vi "SiggenSetFreq.vi"(2 "error in (no error)":errorcluster, 3 "Freq request (GHz)":dbl=2.45 min=0.6 max=3.0 step=0.001 format="%#_9g") -> (0 "Error status":errorcluster, 1 "Freq returned (GHz)":dbl format="%#_10e")   [LabVIEW 2009]
doc: "Sets the frequency on the siggen.\nReads the frequency back from the siggen."
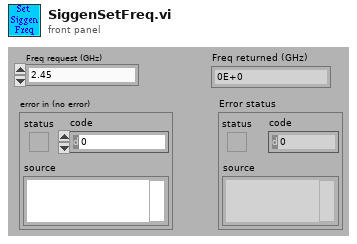
[diagram p1: front panel]
types:
  T1 = enum16{"N1911A", "Siggen", "34980a", "E4418B", "Rvp8"}
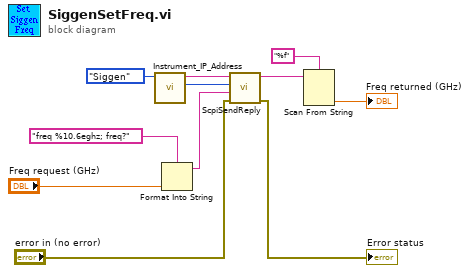
[diagram p0: block diagram]
diagram:
  n1 = call "Instrument_IP_Address.vi"("Instrument"=T1."Siggen") -> ("Port"=w2:u16, "IP Address"=w3:string)  [unwired: 9 in]
  n2 = Format Into String(format string="freq %10.6eghz; freq?", "Freq request (GHz)") -> (resulting string=w8:string)  [unwired: 2 in, 1 out]
  n3 = call "ScpiSendReply.vi"("error in (no error)"="error in (no error)", "Command"=w8, "TCP port"=w2, "IP Address"=w3) -> ("Error out"=→"Error status":errorcluster, "Reply"=w6:string)  [unwired: 5 in]
  n4 = Scan From String(format string="%f", input string=w6) -> (output 1=→"Freq returned (GHz)":dbl)  [unwired: 3 in, 3 out]
